vi "Recieve Data.vi"(8 "error in (no error)":errorcluster, 9 "Force read":bool, 10 "Points to read":i32, 11 "RP Instrument in":refnum<class "RP Instrument.lvclass">) -> (0 "error out":errorcluster, 2 "Data out":i32[](array[numeric]), 3 "RP Instrument out":refnum<class "RP Instrument.lvclass">)   [LabVIEW 2016, in "RP Instrument.lvclass"]
uses:
  RP Instrument.lvclass
  RP Instrument.lvclass/RP Instrument.ctl
  RP Communicator/RP Communicator.lvclass
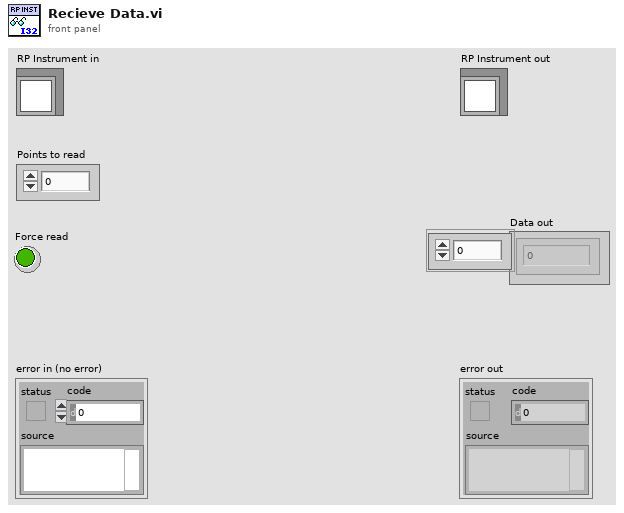
[diagram p1: front panel]
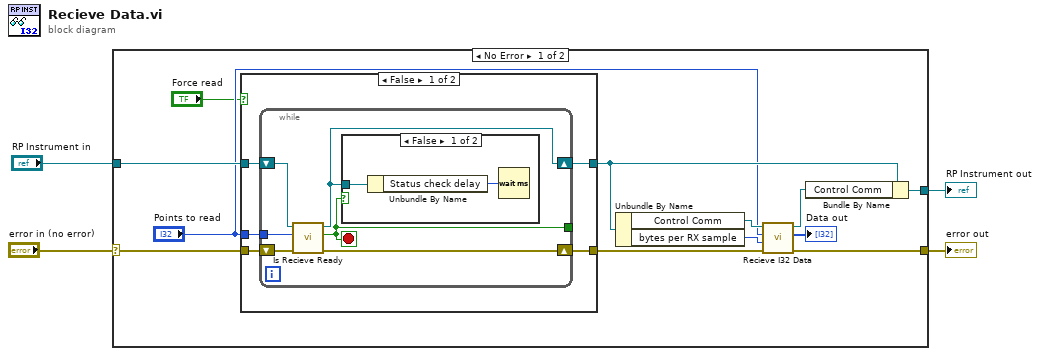
[diagram p0: block diagram]
diagram:
  n1 = case shown="No Error" "error in (no error)" {
    selector: "error in (no error)" -> [w11 w33]
    tunnel: [w12 w33] -> w3
    tunnel: [w13 w32] -> w1
    tunnel: "RP Instrument in" -> [w8 w32]
    frame No Error {
      n2 = case shown="False" "Force read" {
        tunnel: w11 -> [w21 w30]
        tunnel: [w20 w30] -> w10
        tunnel: [w19 w31] -> w9
        tunnel: w8 -> [w18 w31]
        tunnel: "Points to read" -> [w17 _]
        frame False {
          n3 = while {
            shift-right: [w25] -> w20
            shift-left: w21 -> [w26]
            shift-right: [w22] -> w19
            shift-left: w18 -> [w27]
            tunnel: [w24] -> _
            tunnel: w17 -> [w23]
            stop <- w24 stop-if-true
            n4 = call-dynamic "Is Recieve Ready.vi"("error in (no error)"=w26, "Points to read"=w23, "RP Instrument in"=w27) -> ("error out"=w25:errorcluster, "Recieve Ready"=w24:bool, "RP Instrument out"=w22:refnum<class "RP Instrument.lvclass">)  [unwired: 5 in, 1 out]
            n5 = case shown="False" w24 {
              tunnel: w22 -> [w29 _]
              frame False {
                n6 = Unbundle By Name(w29) -> ("Status check delay"=w28:u32)
                n7 = Wait (ms)(milliseconds to wait=w28) -> ()  [unwired: 1 out]
              }
              frame True {
              }
            }
          }
        }
        frame True {
        }
      }
      n8 = Unbundle By Name(w9) -> ("Control Comm"=w14:refnum<class "RP Communicator.lvclass">, "bytes per RX sample"=w6:u32)
      n9 = call-dynamic "Recieve I32 Data.vi"("error in (no error)"=w10, "bytes per sample"=w6, "Samples per read"="Points to read", "RP Communicator in"=w14) -> ("error out"=w12:errorcluster, "Data out"=→"Data out":i32[], "RP Communicator out"=w15:refnum<class "RP Communicator.lvclass">)  [unwired: 5 in]
      n10 = Bundle By Name(cluster=w9, "Control Comm"=w15) -> (w13:refnum<class "RP Instrument.lvclass">)
    }
    frame Error {
    }
  }
  "error out" <- w3
  "RP Instrument out" <- w1
